vi "RSZVB Additional Directory Calibration Kit.vi"(8 "error in (no error)":errorcluster {"code" format="%.0x"}, 10 "Directory":string, 11 "VISA session":refnum<visa-resource-name>) -> (0 "error out":errorcluster {"code" format="%.0x"}, 3 "dup VISA session":refnum<visa-resource-name>)   [LabVIEW 2011]
doc: "This VI specifies the Directory for Additionally Available Cal Kits and Conn Types. All cal kit files in the special directory will be (re-)loaded automatically every time the NWA application is started.\n\n\nRemote-control command(s):\nMMEMory:LOAD:CKIT:UDIRectory '<directory>'"
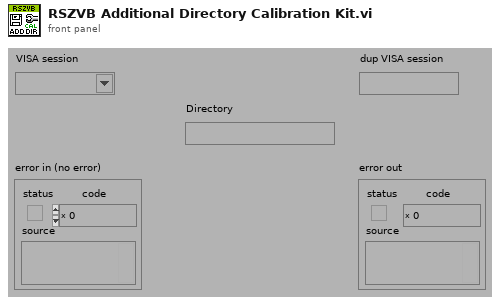
[diagram p1: front panel]
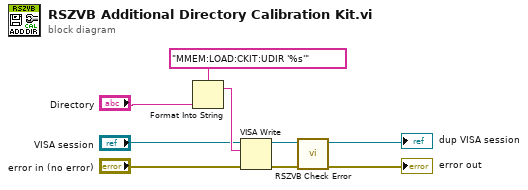
[diagram p0: block diagram]
diagram:
  n1 = Format Into String(format string="MMEM:LOAD:CKIT:UDIR '%s'", "Directory") -> (resulting string=w6:string)  [unwired: 2 in, 1 out]
  n2 = VISA Write(VISA resource name="VISA session", write buffer=w6, error in (no error)="error in (no error)") -> (VISA resource name out=w7:refnum<visa-resource-name>, error out=w8:errorcluster)  [unwired: 1 out]
  n3 = call "RSZVB Check Error.vi"("error in (no error)"=w8, "VISA session"=w7) -> ("error out"=→"error out":errorcluster, "dup VISA session"=→"dup VISA session":refnum<visa-resource-name>)  [unwired: 8 in]
